vi "fgv_cam.vi"(7 "cmd":enum16{"ini", "grab", "close", "read"}(ring), 8 "error in":errorcluster, 11 "Image In":T1) -> (0 "error out":errorcluster, 2 "Session Out":T2, 3 "Image Out":T1)   [LabVIEW 2019]
uses:
  <vilib>/userDefined/High Color/IMAQdx.ctl
  <vilib>/vision/Image Controls.llb/IMAQ Image.ctl
  <vilib>/vision/driver/IMAQdx.llb/IMAQdx Buffer Number Mode.ctl
  <vilib>/vision/driver/NI_Vision_Acquisition_Software.lvlib
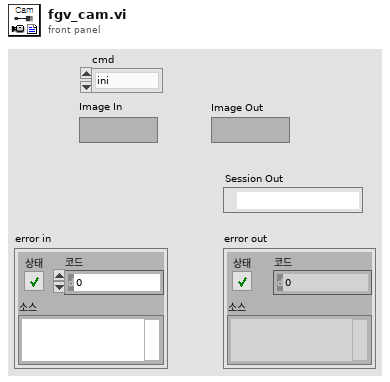
[diagram p1: front panel]
types:
  T1 = typedef "IMAQ Image.ctl" = refnum<image>
  T2 = typedef "IMAQdx.ctl" = refnum<k21>
  T3 = typedef "NI_Vision_Acquisition_Software.lvlib/IMAQdx Buffer Number Mode.ctl" = enum32{"Next", "Last", "Buffer Number", "Every", "Last New"}
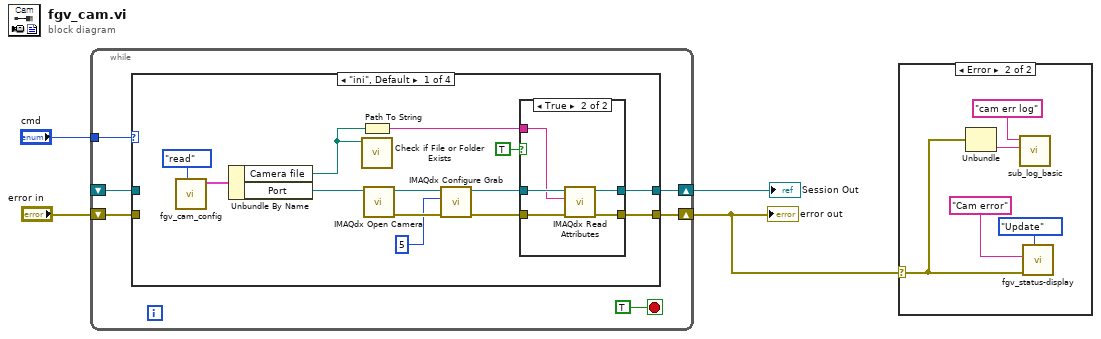
[diagram p0: block diagram]
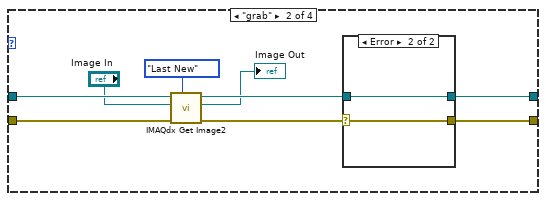
[diagram p4: hidden frame]
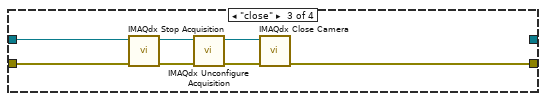
[diagram p6: hidden frame]
diagram:
  n1 = while {
    tunnel: "cmd" -> [w9]
    shift-right: [w7] -> w1
    shift-left: "error in" -> [w8]
    shift-right: [w6] -> w2
    shift-left: _ -> [w5]
    stop <- TRUE stop-if-true
    n2 = case shown="\"ini\", Default" w9 {
      tunnel: w8 -> [_ w38 w46 w52]
      tunnel: [w12 w36 w50 w52] -> w7
      tunnel: [w13 w35 _ w51] -> w6
      tunnel: w5 -> [_ w39 w47 w51]
      frame "ini", Default {
        n3 = call "fgv_cam_config.vi"("cmd"=enum16{"read", "write"}."read") -> ("camera cfg out"=w21:cluster{"Port":T2, "Camera file":path})  [unwired: 10 in]
        n4 = Unbundle By Name(w21) -> ("Camera file"=w19:path, "Port"=w20:T2)
        n5 = Path To String(path=w19) -> (string=w23:string)
        n6 = call <vilib>:"Check if File or Folder Exists.vi"("path"=w19) -> ()  [unwired: 8 in, 3 out]
        n7 = call <vilib>:"IMAQdx Open Camera.vi"("Session In"=w20) -> ("error out"=w17:errorcluster, "Session Out"=w18:T2)  [unwired: 9 in]
        n8 = call <vilib>:"IMAQdx Configure Grab.vi"("error in"=w17, "Number of Buffers"=u32 5, "Session In"=w18) -> ("error out"=w15:errorcluster, "Session Out"=w16:T2)  [unwired: 7 in]
        n9 = case shown="True" TRUE {
          tunnel: [w25 w30] -> w13
          tunnel: [w24 w29] -> w12
          tunnel: w16 -> [w25 w28]
          tunnel: w15 -> [w24 w27]
          tunnel: w23 -> [_ w26]
          frame False {
          }
          frame True {
            n10 = call <vilib>:"IMAQdx Read Attributes.vi"("error in"=w27, "Filename"=w26, "Session In"=w28) -> ("error out"=w29:errorcluster, "Session Out"=w30:T2)  [unwired: 7 in]
          }
        }
      }
      frame "grab" {
        n11 = call <vilib>:"IMAQdx Get Image2.vi"("Buffer Number Mode (Next)"=IMAQdx_Buffer_Number_Mode."Last New", "error in"=w38, "Image In"="Image In", "Session In"=w39) -> ("error out"=w37:errorcluster, "Image Out"=→"Image Out":T1, "Session Out"=w34:T2)  [unwired: 4 in, 1 out]
        n12 = case shown="Error" w37 {
          selector: w37 -> [w41 w43]
          tunnel: [w41 w43] -> w36
          tunnel: [w40 w42] -> w35
          tunnel: w34 -> [w40 w42]
          frame No Error {
          }
          frame Error {
          }
        }
      }
      frame "close" {
        n13 = call <vilib>:"IMAQdx Stop Acquisition.vi"("error in"=w46, "Session In"=w47) -> ("error out"=w48:errorcluster, "Session Out"=w49:T2)  [unwired: 8 out]
        n14 = call <vilib>:"IMAQdx Unconfigure Acquisition.vi"("error in"=w48, "Session In"=w49) -> ("error out"=w44:errorcluster, "Session Out"=w45:T2)  [unwired: 8 out]
        n15 = call <vilib>:"IMAQdx Close Camera.vi"("error in"=w44, "Session In"=w45) -> ("error out"=w50:errorcluster)  [unwired: 9 in]
      }
      frame "read" {
      }
    }
  }
  "error out" <- w1
  "Session Out" <- w2
  n16 = case shown="Error" w1 {
    selector: w1 -> [_ w53]
    frame No Error {
    }
    frame Error {
      n17 = Unbundle(w53) -> ("source"=w54:string)  [unwired: 2 out]
      n18 = call "sub_log_basic.vi"("desc"=w54, "Title"="cam err log") -> ()  [unwired: 9 in, 1 out]
      n19 = call "fgv_status-display.vi"("Mode"=enum16{"Initial", "Update", "Clear"}."Update", "error in"=w53, "title"="Cam error" ("String in")) -> ()  [unwired: 8 in, 1 out]
    }
  }
